vi "Set InvokeReponse.vi"(8 "error in (no error)":errorcluster, 10 "InvokeResponse_Data":T1, 11 "gRPCid":T2) -> (0 "error out":errorcluster)   [LabVIEW 2019, in "OOP Server.lvclass"]
uses:
  OOP Server.lvclass
  gRPC interface/Server API/typeDefs/grpcId.ctl
  InvokeResponse_Data.ctl
  dcc74a39-081a-4bdd-860b-8ed792803c96.vi
  <vilib>/Utility/error.llb/Error Cluster From Error Code.vi
  gRPC interface/gprc-lvsupport.lvlib
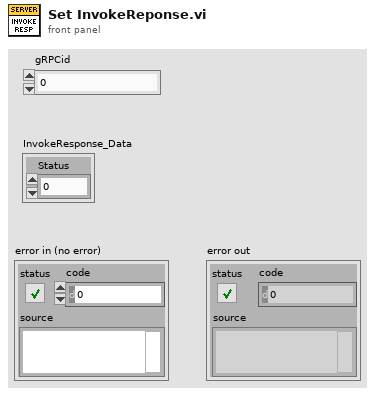
[diagram p1: front panel]
types:
  T1 = typedef "OOP Server.lvclass/InvokeResponse_Data.ctl" = cluster{"Status":i32}
  T2 = typedef "gprc-lvsupport.lvlib/grpcId.ctl" = u64
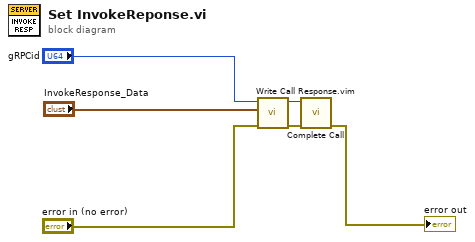
[diagram p0: block diagram]
diagram:
  n1 = call "Write Call Response.vim"("error in (no error)"="error in (no error)", "Response Data"="InvokeResponse_Data", "gRPCid in"="gRPCid") -> ("error out"=w3:errorcluster, "gRPCid"=w4:T2)  [unwired: 7 in]
  n2 = call "Complete Call.vi"("gRPCid"=w4, "error in (no error)"=w3) -> ("error out"=→"error out":errorcluster)  [unwired: 8 in]
